vi "DAQ.EnumerateAndSortDevices.vi"(8 "error in (no error)":errorcluster, 11 "Instrument.DAQ":refnum<class "Instrument.DAQ.lvclass">) -> (0 "error out":errorcluster, 2 "Devices (sorted)":T1[](array[typedef])=[{"DeviceName"="PXI1Slot5", "DevIsSimulated"=FALSE, "DeviceSerialNumber"=21267641, "ProductType"="PXI-4461", "ProductCategory"=14649, "ProductNumber"=29299, "ChassisNumber"=1, "SlotNumber"=5, "ChassisName"="NI PXIe-1082DC", "ChassisSerialNumber"=50979316}, {"DeviceName"="PXI1Slot6", "DevIsSimulated"=FALSE, "DeviceSerialNumber"=21267639, "ProductType"="PXI-4461", "ProductCategory"=14649, "ProductNumber"=29299, "ChassisNumber"=1, "SlotNumber"=6, "ChassisName"="NI PXIe-1082DC", "ChassisSerialNumber"=50979316}, {"DeviceName"="PXI1Slot7", "DevIsSimulated"=FALSE, "DeviceSerialNumber"=20037036, "ProductType"="PXI-4461", "ProductCategory"=14649, "ProductNumber"=29299, "ChassisNumber"=1, "SlotNumber"=7, "ChassisName"="NI PXIe-1082DC", "ChassisSerialNumber"=50979316}, {"DeviceName"="PXI1Slot8", "DevIsSimulated"=FALSE, "DeviceSerialNumber"=20037044, "ProductType"="PXI-4461", "ProductCategory"=14649, "ProductNumber"=29299, "ChassisNumber"=1, "SlotNumber"=8, "ChassisName"="NI PXIe-1082DC", "ChassisSerialNumber"=50979316}, {"DeviceName"="Dev1", "DevIsSimulated"=FALSE, "DeviceSerialNumber"=0, "ProductType"="", "ProductCategory"=0, "ProductNumber"=0, "ChassisNumber"=4294967295, "SlotNumber"=0, "ChassisName"="", "ChassisSerialNumber"=0}], 3 "Instrument.DAQ out":refnum<class "Instrument.DAQ.lvclass">)   [LabVIEW 2019, in "Instrument.Lockin.lvlib" / "Instrument.DAQ.lvclass"]
uses:
  Instrument.DAQ.lvclass
  Typedefs/DeviceInfo--Cluster.ctl
  Instrument.DAQ.lvclass/Instrument.DAQ.ctl
  <userlib>/_OpenG.lib/array/array.llb/Sort 1D Array (U32)__ogtk.vi
  <userlib>/_OpenG.lib/array/array.llb/Reorder 1D Array2 (Variant)__ogtk.vi
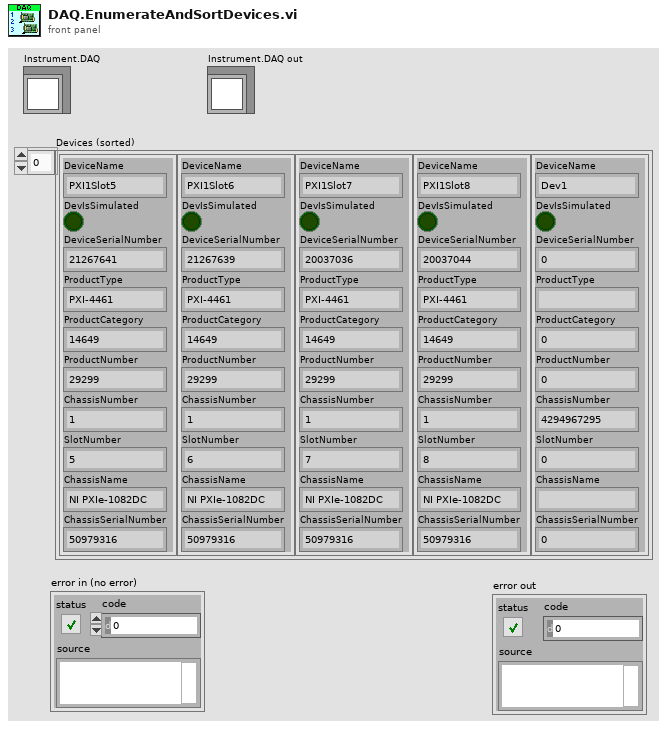
[diagram p1: front panel]
types:
  T1 = typedef "Instrument.Lockin.lvlib/Instrument.DAQ.lvclass/DeviceInfo--Cluster.ctl" = cluster{"DeviceName":string, "DevIsSimulated":bool, "DeviceSerialNumber":u32, "ProductType":string, "ProductCategory":i32, "ProductNumber":u32, "ChassisNumber":u32, "SlotNumber":u32, "ChassisName":string, "ChassisSerialNumber":u32}
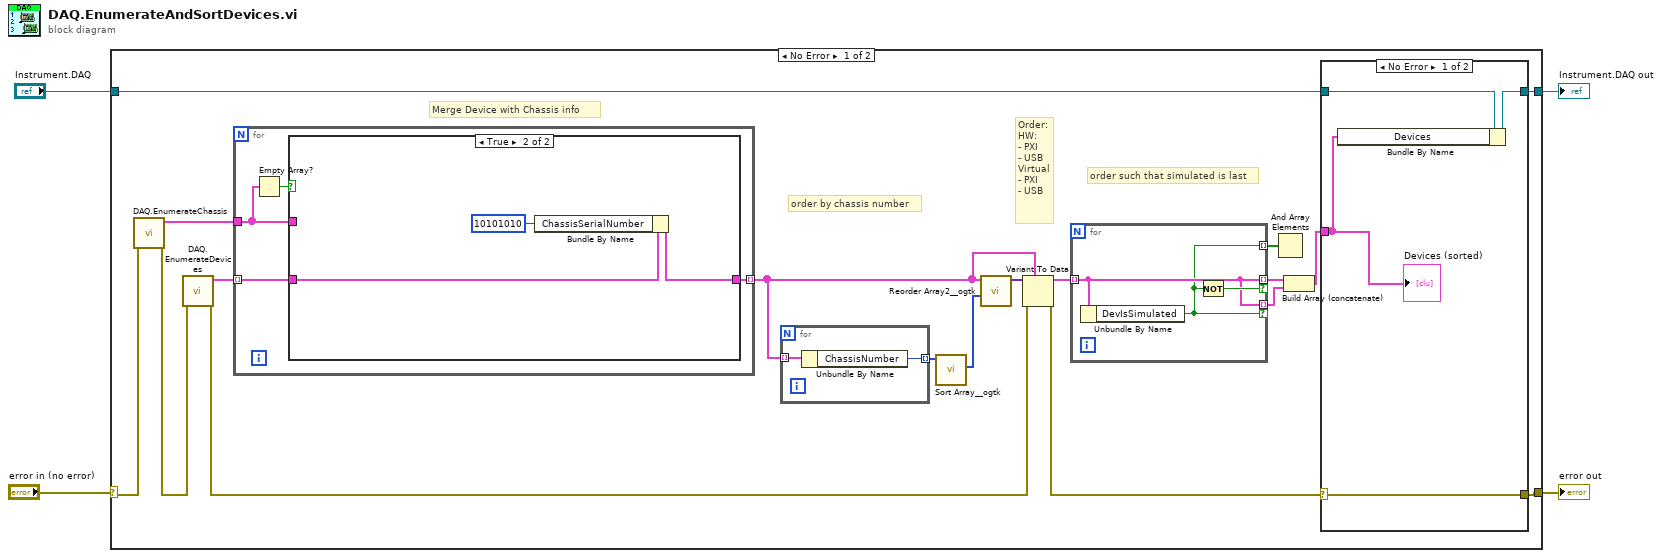
[diagram p0: block diagram]
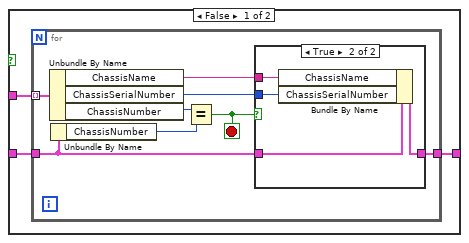
[diagram p2: hidden frame]
diagram:
  n1 = case shown="No Error" "error in (no error)" {
    selector: "error in (no error)" -> [w7 w58]
    tunnel: [w13 w58] -> w3
    tunnel: "Instrument.DAQ" -> [w10 w57]
    tunnel: [w11 w57] -> w1
    frame No Error {
      # "Order:\nHW:\n- PXI\n- USB\nVirtual\n- PXI\n- USB"
      # "order by chassis number"
      # "order such that simulated is last"
      # "Merge Device with Chassis info"
      n2 = call "DAQ.EnumerateChassis.vi"("error in (no error)"=w7) -> ("error out"=w6:errorcluster, "Chassis"=w19:T1[])  [unwired: 9 in]
      n3 = call "DAQ.EnumerateDevices.vi"("error in (no error)"=w6) -> ("error out"=w5:errorcluster, "Devices"=w20:T1[])  [unwired: 9 in]
      n4 = for {
        tunnel: w19 -> [w24]
        tunnel: w20 -> [w25] mode=indexing
        tunnel: [w26] -> w15 mode=indexing
        n5 = Empty Array?(array=w24) -> (empty?=w23:bool)
        n6 = case shown="True" w23 {
          tunnel: [w29 w45] -> w26
          tunnel: w25 -> [w28 w44]
          tunnel: w24 -> [w27 _]
          frame False {
            n7 = for {
              tunnel: w28 -> [w30]
              tunnel: w27 -> [w37] mode=indexing
              tunnel: [w32] -> w29
              stop <- w31 stop-if-true
              n8 = Unbundle By Name(w37) -> ("ChassisName"=w34:string, "ChassisSerialNumber"=w33:u32, "ChassisNumber"=w36:u32)
              n9 = Unbundle By Name(w30) -> ("ChassisNumber"=w35:u32)
              n10 = Equal?(x=w36, y=w35) -> (x = y?=w31:bool)
              n11 = case shown="True" w31 {
                tunnel: w30 -> [w38 w42]
                tunnel: w34 -> [_ w41]
                tunnel: w33 -> [_ w39]
                tunnel: [w38 w40] -> w32
                frame False {
                }
                frame True {
                  n12 = Bundle By Name(cluster=w42, "ChassisName"=w41, "ChassisSerialNumber"=w39) -> (w40:T1)
                }
              }
            }
          }
          frame True {
            n13 = Bundle By Name(cluster=w44, "ChassisSerialNumber"=u32 10101010) -> (w45:T1)
          }
        }
      }
      n14 = for {
        tunnel: w15 -> [w50] mode=indexing
        tunnel: [w49] -> w18 mode=indexing
        n15 = Unbundle By Name(w50) -> ("ChassisNumber"=w49:u32)
      }
      n16 = call-poly <userlib>:"Sort Array__ogtk.vi"("Array in"=w18) -> ("Sorted Pointers"=w17:i32[])  [unwired: 9 in, 1 out]
      n17 = call-poly <userlib>:"Reorder Array2__ogtk.vi"("indices"=w17, "array"=w15) -> ("reordered array"=w16:variant[])  [unwired: 9 in]
      n18 = Variant To Data(error in=w5, type=w15, Variant=w16) -> (data=w14:T1[], error out=w12:errorcluster)
      n19 = for {
        tunnel: [w47] -> w22 mode=indexing if=w48
        tunnel: w14 -> [w47] mode=indexing
        tunnel: [w47] -> w21 mode=indexing if=w46
        tunnel: [w46] -> w9 mode=indexing
        n20 = Unbundle By Name(w47) -> ("DevIsSimulated"=w46:bool)
        n21 = Not(x=w46) -> (.not. x?=w48:bool)
      }
      n22 = And Array Elements(Boolean array=w9) -> ()  [unwired: 1 out]
      n23 = Build Array (concatenate)(w22, w21) -> (w8:T1[])
      n24 = case shown="No Error" w12 {
        selector: w12 -> [w54 w55]
        tunnel: [w54 w55] -> w13
        tunnel: [w52 w56] -> w11
        tunnel: w10 -> [w53 w56]
        tunnel: w8 -> [w51 _]
        frame No Error {
          n25 = Bundle By Name(cluster=w53, "Devices"=w51) -> (w52:refnum<class "Instrument.DAQ.lvclass">)
          "Devices (sorted)" <- w51
        }
        frame Error {
        }
      }
    }
    frame Error {
    }
  }
  "error out" <- w3
  "Instrument.DAQ out" <- w1
